vi "Configure FPGA ADXL345.vi"(11 "Private Data In":T1) -> (3 "Private Data Out":T1)   [LabVIEW 2014]
uses:
  <vilib>/IEDriver/SPIandI2C/FPGA/Type Def/Private Data (SPI).ctl
  <vilib>/IEDriver/SPIandI2C/FPGA/Library/IP SPI&I2C.lvlib
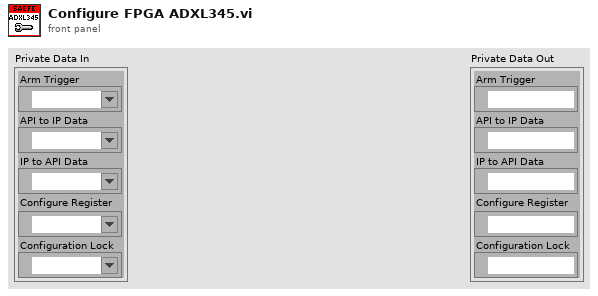
[diagram p1: front panel]
types:
  T1 = typedef "IP SPI&I2C.lvlib/Private Data (SPI).ctl" = cluster{"Arm Trigger":refnum<k21>, "API to IP Data":refnum<k21>, "IP to API Data":refnum<k21>, "Configure Register":refnum<k21>, "Configuration Lock":refnum<k21>}
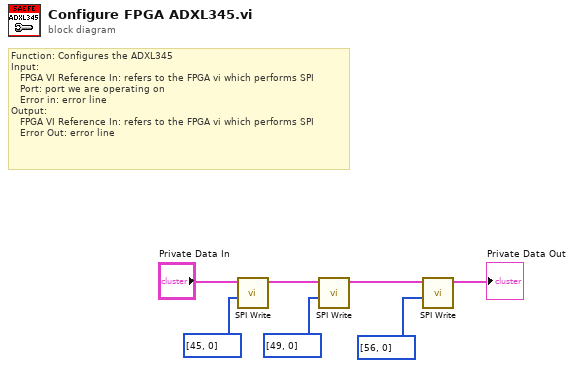
[diagram p0: block diagram]
diagram:
  # "Function: Configures the ADXL345\nInput:\n   FPGA VI Reference In: refers to the FPGA vi which performs SPI\n   Port: port we are operating on\n   Error in: error line\nOutput:\n   FPGA VI Reference In: refers to the FPGA vi which performs SPI\n   Error Out: error line"
  n1 = call "SPI Write.vi"("Write Data"=u8[] [45, 0], "Private Data In"="Private Data In") -> ("Private Data Out"=w7:T1)  [unwired: 8 in, 1 out]
  n2 = call "SPI Write.vi"("Write Data"=u8[] [49, 0], "Private Data In"=w7) -> ("Private Data Out"=w6:T1)  [unwired: 8 in, 1 out]
  n3 = call "SPI Write.vi"("Write Data"=u8[] [56, 0], "Private Data In"=w6) -> ("Private Data Out"=→"Private Data Out":T1)  [unwired: 8 in, 1 out]
